vi "8-2.vi"() -> ()   [LabVIEW 2019, in "8.lvlib"]
uses:
  8.lvlib
panel:
  out "decodes":i32[](array[numeric]) format="%04.0f"
  out "Sum of decodes":i32
  out "codes":string[][](array[string])
  out "patterns":string[][](array[string])
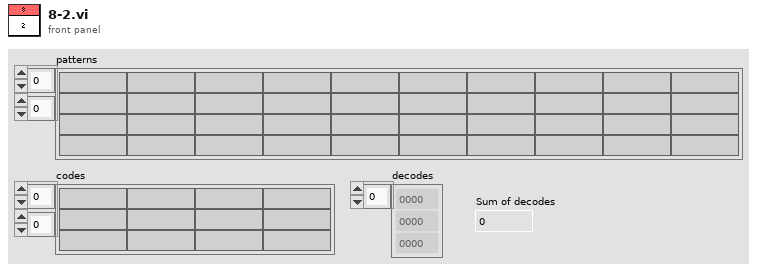
[diagram p1: front panel]
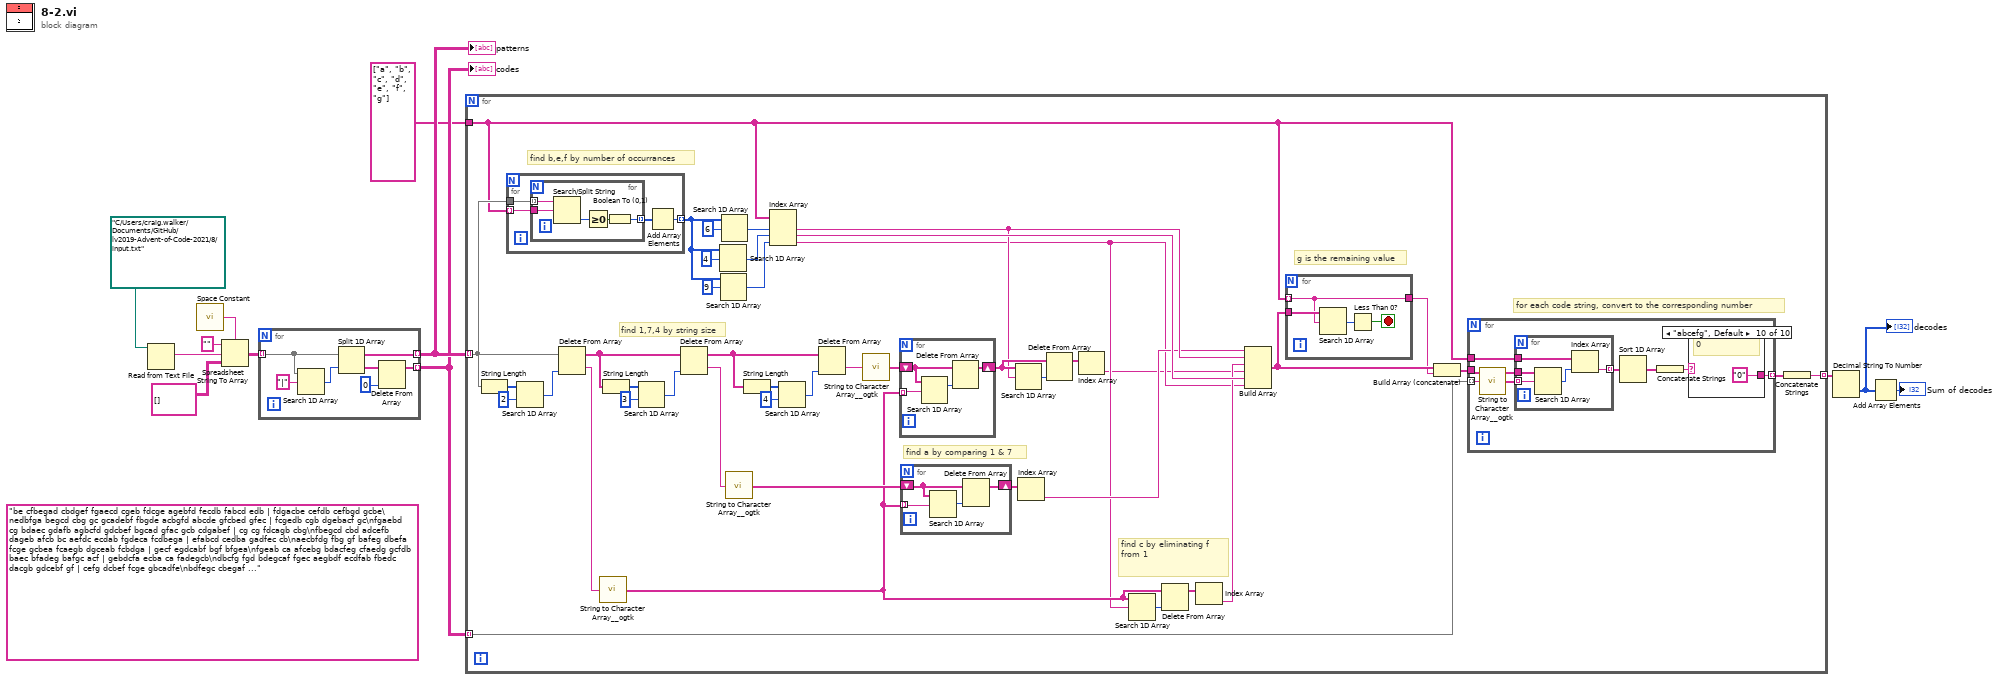
[diagram p0: block diagram]
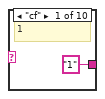
[diagram p2: hidden frame]
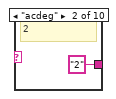
[diagram p3: hidden frame]
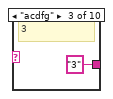
[diagram p4: hidden frame]
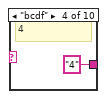
[diagram p5: hidden frame]
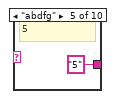
[diagram p6: hidden frame]
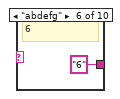
[diagram p7: hidden frame]
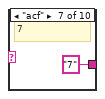
[diagram p8: hidden frame]
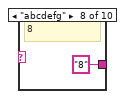
[diagram p9: hidden frame]
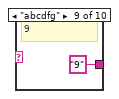
[diagram p10: hidden frame]
diagram:
  (unwired) "be cfbegad cbdgef fgaecd cgeb fdcge agebfd fecdb fabcd edb | fdgacbe cefdb cefbgd gcbe\nedbfga begcd cbg gc gcadebf fbgde acbgfd abcde gfcbed gfec | fcgedb cgb dgebacf gc\nfgaebd cg bdaec gdafb agbcfd gdcbef bgcad gfac gcb cdgabef | cg cg fdcagb cbg\nfbegcd cbd adcefb dageb afcb bc aefdc ecdab fgdeca fcdbega | efabcd cedba gadfec cb\naecbfdg fbg gf bafeg dbefa fcge gcbea fcaegb dgceab fcbdga | gecf egdcabf bgf bfgea\nfgeab ca afcebg bdacfeg cfaedg gcfdb baec bfadeg bafgc acf | gebdcfa ecba ca fadegcb\ndbcfg fgd bdegcaf fgec aegbdf ecdfab fbedc dacgb gdcebf gf | cefg dcbef fcge gbcadfe\nbdfegc cbegaf gecbf dfcage bdacg ed bedf ced adcbefg gebcd | ed bcgafe cdgba cbgef\negadfb cdbfeg cegd fecab cgb gbdefca cg fgcdab egfdb bfceg | gbdfcae bgc cg cgb\ngcafb gcf dcaebfg ecagb gf abcdeg gaef cafbge fdbac fegbdc | fgae cfgab fg bagce" ("element")
  n1 = Read from Text File(file (use dialog)=path "C:/Users/craig.walker/Documents/GitHub/lv2019-Advent-of-Code-2021/8/input.txt") -> (text=w1:string)  [unwired: 3 in, 3 out]
  n2 = call <vilib>:"Space Constant.vi"() -> ("String"=w10:string)
  n3 = Spreadsheet String To Array(delimiter (Tab)=w10, format string="", spreadsheet string=w1, array type (2D Dbl)=string[][] []) -> (array=w11:string[][])
  n4 = for {
    tunnel: w11 -> [w15] mode=indexing
    tunnel: [w14] -> w6 mode=indexing
    tunnel: [w13] -> w7 mode=indexing
    n5 = Search 1D Array(1D array=w15, element="|") -> (index of element=w18:i32)  [unwired: 1 in]
    n6 = Split 1D Array(array=w15, index=w18) -> (first subarray=w13:string[], second subarray=w17:string[])
    n7 = Delete From Array(array=w17, index=0) -> (array with subset deleted=w14:string[])  [unwired: 1 in, 1 out]
  }
  "patterns" <- w7
  "codes" <- w6
  n8 = for {
    tunnel: w7 -> [w51] mode=indexing
    tunnel: w6 -> [w36] mode=indexing
    tunnel: string[] ["a", "b", "c", "d", "e", "f", "g"] -> [w34]
    tunnel: [w32] -> w4 mode=indexing
    # "for each code string, convert to the corresponding number"
    # "g is the remaining value"
    # "find a by comparing 1 & 7"
    # "find b,e,f by number of occurrances"
    # "find 1,7,4 by string size"
    # "find c by eliminating f from 1"
    n9 = String Length(string=w51) -> (length=w62:i32[])
    n10 = for {
      tunnel: w51 -> [w71]
      tunnel: w34 -> [w70] mode=indexing
      tunnel: [w68] -> w46 mode=indexing
      n11 = for {
        tunnel: w71 -> [w76] mode=indexing
        tunnel: w70 -> [w75]
        tunnel: [w72] -> w69 mode=indexing
        n12 = Search/Split String(string=w76, search string/char (-)=w75) -> (offset of match=w74:i32)  [unwired: 1 in, 2 out]
        n13 = Greater Or Equal To 0?(x=w74) -> (x >= 0?=w73:bool)
        n14 = Boolean To (0,1)(Boolean=w73) -> (0, 1=w72:i16)
      }
      n15 = Add Array Elements(numeric array=w69) -> (sum=w68:i16)
    }
    n16 = Search 1D Array(1D array=w62, element=2) -> (index of element=w63:i32)  [unwired: 1 in]
    n17 = Delete From Array(array=w51, index=w63) -> (deleted portion=w56:string, array with subset deleted=w57:string[])  [unwired: 1 in]
    n18 = call <userlib>:"String to Character Array__ogtk.vi"("Input String"=w56) -> ("Character Array"=w22:string[])
    n19 = String Length(string=w57) -> (length=w59:i32[])
    n20 = Search 1D Array(1D array=w59, element=3) -> (index of element=w58:i32)  [unwired: 1 in]
    n21 = Delete From Array(array=w57, index=w58) -> (deleted portion=w31:string, array with subset deleted=w52:string[])  [unwired: 1 in]
    n22 = Search 1D Array(1D array=w46, element=i16 4) -> (index of element=w47:i32)  [unwired: 1 in]
    n23 = Search 1D Array(1D array=w46, element=i16 9) -> (index of element=w44:i32)  [unwired: 1 in]
    n24 = Search 1D Array(1D array=w46, element=i16 6) -> (index of element=w49:i32)  [unwired: 1 in]
    n25 = call <userlib>:"String to Character Array__ogtk.vi"("Input String"=w31) -> ("Character Array"=w30:string[])
    n26 = String Length(string=w52) -> (length=w54:i32[])
    n27 = Index Array(array=w34, index #1=w49, index #2=w47, index #3=w44) -> (element #1=w25:string, element #2=w39:string, element #3=w21:string)
    n28 = Search 1D Array(1D array=w54, element=4) -> (index of element=w55:i32)  [unwired: 1 in]
    n29 = Delete From Array(array=w52, index=w55) -> (deleted portion=w28:string)  [unwired: 1 in, 1 out]
    n30 = call <userlib>:"String to Character Array__ogtk.vi"("Input String"=w28) -> ("Character Array"=w27:string[])
    n31 = for {
      tunnel: w22 -> [w79] mode=indexing
      shift-right: [w77] -> w26
      shift-left: w27 -> [w78]
      n32 = Search 1D Array(1D array=w78, element=w79) -> (index of element=w80:i32)  [unwired: 1 in]
      n33 = Delete From Array(array=w78, index=w80) -> (array with subset deleted=w77:string[])  [unwired: 1 in, 1 out]
    }
    n34 = for {
      tunnel: w22 -> [w84] mode=indexing
      shift-right: [w81] -> w29
      shift-left: w30 -> [w82]
      n35 = Search 1D Array(1D array=w82, element=w84) -> (index of element=w83:i32)  [unwired: 1 in]
      n36 = Delete From Array(array=w82, index=w83) -> (array with subset deleted=w81:string[])  [unwired: 1 in, 1 out]
    }
    n37 = Search 1D Array(1D array=w26, element=w25) -> (index of element=w42:i32)  [unwired: 1 in]
    n38 = Index Array(array=w29) -> (element=w24:string)  [unwired: 1 in]
    n39 = Delete From Array(array=w26, index=w42) -> (array with subset deleted=w40:string[])  [unwired: 1 in, 1 out]
    n40 = Index Array(array=w40) -> (element=w20:string)  [unwired: 1 in]
    n41 = Search 1D Array(1D array=w22, element=w21) -> (index of element=w43:i32)  [unwired: 1 in]
    n42 = Delete From Array(array=w22, index=w43) -> (array with subset deleted=w41:string[])  [unwired: 1 in, 1 out]
    n43 = Index Array(array=w41) -> (element=w23:string)  [unwired: 1 in]
    n44 = Build Array(w24, w25, w23, w20, w39, w21) -> (w38:string[])
    n45 = for {
      tunnel: w34 -> [w65] mode=indexing
      tunnel: w38 -> [w67]
      tunnel: [w65] -> w37
      stop <- w64 stop-if-true
      n46 = Search 1D Array(1D array=w67, element=w65) -> (index of element=w66:i32)  [unwired: 1 in]
      n47 = Less Than 0?(x=w66) -> (x < 0?=w64:bool)
    }
    n48 = Build Array (concatenate)(w38, w37) -> (w35:string[])
    n49 = for {
      tunnel: [w92] -> w33 mode=indexing
      tunnel: w36 -> [w91] mode=indexing
      tunnel: w35 -> [w90]
      tunnel: w34 -> [w88]
      n50 = call <userlib>:"String to Character Array__ogtk.vi"("Input String"=w91) -> ("Character Array"=w89:string[])
      n51 = for {
        tunnel: w90 -> [w97]
        tunnel: w89 -> [w96] mode=indexing
        tunnel: w88 -> [w95]
        tunnel: [w93] -> w87 mode=indexing
        n52 = Search 1D Array(1D array=w97, element=w96) -> (index of element=w94:i32)  [unwired: 1 in]
        n53 = Index Array(array=w95, index=w94) -> (element=w93:string)
      }
      n54 = Sort 1D Array(array=w87) -> (sorted array=w85:string[])
      n55 = Concatenate Strings(w85) -> (w86:string)
      n56 = case shown="\"abcefg\", Default" w86 {
        tunnel: ["1" "2" "3" "4" "5" "6" "7" "8" "9" "0"] -> w92
        frame "cf" {
          # "1"
        }
        frame "acdeg" {
          # "2"
        }
        frame "acdfg" {
          # "3"
        }
        frame "bcdf" {
          # "4"
        }
        frame "abdfg" {
          # "5"
        }
        frame "abdefg" {
          # "6"
        }
        frame "acf" {
          # "7"
        }
        frame "abcdefg" {
          # "8"
        }
        frame "abcdfg" {
          # "9"
        }
        frame "abcefg", Default {
          # "0"
        }
      }
    }
    n57 = Concatenate Strings(w33) -> (w32:string)
  }
  n58 = Decimal String To Number(string=w4) -> (number=w3:i32[])  [unwired: 2 in, 1 out]
  "decodes" <- w3
  n59 = Add Array Elements(numeric array=w3) -> (sum=→"Sum of decodes":i32)
